vi "StopOnSightProportional.vi"() -> ()   [LabVIEW 2013]
uses:
  <vilib>/Platform/TimedLoop/XDataNode/timing_clust.ctl
  <vilib>/Platform/TimedLoop/XDataNode/nitl_modes.ctl
  <vilib>/Platform/TimedLoop/XDataNode/wakeup.ctl
  <vilib>/Instr/_visa.llb/VISA Configure Serial Port (Instr).vi
  <vilib>/FPGAPlugInAG/sbRIO-9642/niLvFpga_Open_sbRIO-9642.vi
  <vilib>/rvi/interface/common/dynamic/niFpgaDynamicAddResources.vi
  <vilib>/rvi/interface/common/niFpgaWaitOnOcc.vi
  <vilib>/Utility/error.llb/Error Cluster From Error Code.vi
  <vilib>/rvi/errors/niLvFpgaAdjustHostInterfaceError.vi
  <vilib>/Platform/TimedLoop/XDataNode/XDataNode.xnode
  <vilib>/rvi/interface/nirviOpenFPGA/nirviOpenFPGA.xnode
  FPGA Bitfiles/NatesProject1_FPGATarget_FPGAConfig_gDHlPw7zMRU.lvbitx
  FPGA Config.vi
  <vilib>/rvi/interface/nirviReadWriteControl/nirviReadWriteControl.xnode
  <vilib>/Platform/TimedLoop/XDataNode/XDNodeRunTimeDep.lvlib
  NiFpgaLv.dll
  <vilib>/rvi/interface/Simulation/niFpgaSimulationCallBeginRW.vi
panel:
  in  "Stop Distance":dbl(slide) scale=0.1..1.5
  out "error out":errorcluster
  out "Distance\n(cm)":dbl(slide) scale=0.0..1.5
  out "ModA/AI0":fxp<+/-,26,5>
  in  "VISA resource name":refnum<visa-resource-name>
  in  "stop":bool
  out "write buffer":string
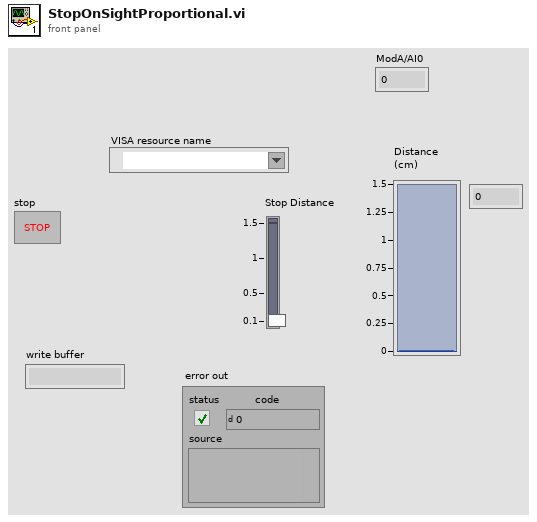
[diagram p1: front panel]
types:
  T1 = typedef "XDNodeRunTimeDep.lvlib/timing_clust.ctl" = cluster{"Expected End [f-1]":u64, "Actual End [f-1]":u64, "Finished Late? [f-1]":bool, "Expected End [i-1]":u64, "Actual End [i-1]":u64, "Finished Late? [i-1]":bool, "Expected Start [i]":u64, "Actual Start [i]":u64, "Expected Start [f]":u64, "Actual Start [f]":u64, "Source Name":string, "Structure Name":string, "Period":i64, "Deadline":i64, "Offset":i64, "Start":i64, "Priority":i32, "Timeout":i32, "Mode":T2, "Wakeup Reason":T3, "Error":errorcluster, "Source Type":string, "Secondary Source Type":string, "Global End Time":u64, "Global Start Time":u64, "Frame Duration":u64, "Iteration Duration":u64, "Assigned CPU":i32, "I/O Scan Engine Mode":u32}
  T2 = typedef "XDNodeRunTimeDep.lvlib/nitl_modes.ctl" = enum32{"No Change", "Process missed periods, maintain original phase", "Discard missed periods, maintain original phase", "Process missed periods, ignore original phase", "Discard missed periods, ignore original phase"}
  T3 = typedef "XDNodeRunTimeDep.lvlib/wakeup.ctl" = enum32{"Normal", "Aborted", "Asynchronous wakeup", "Timing source error", "Timed loop error", "Timeout"}
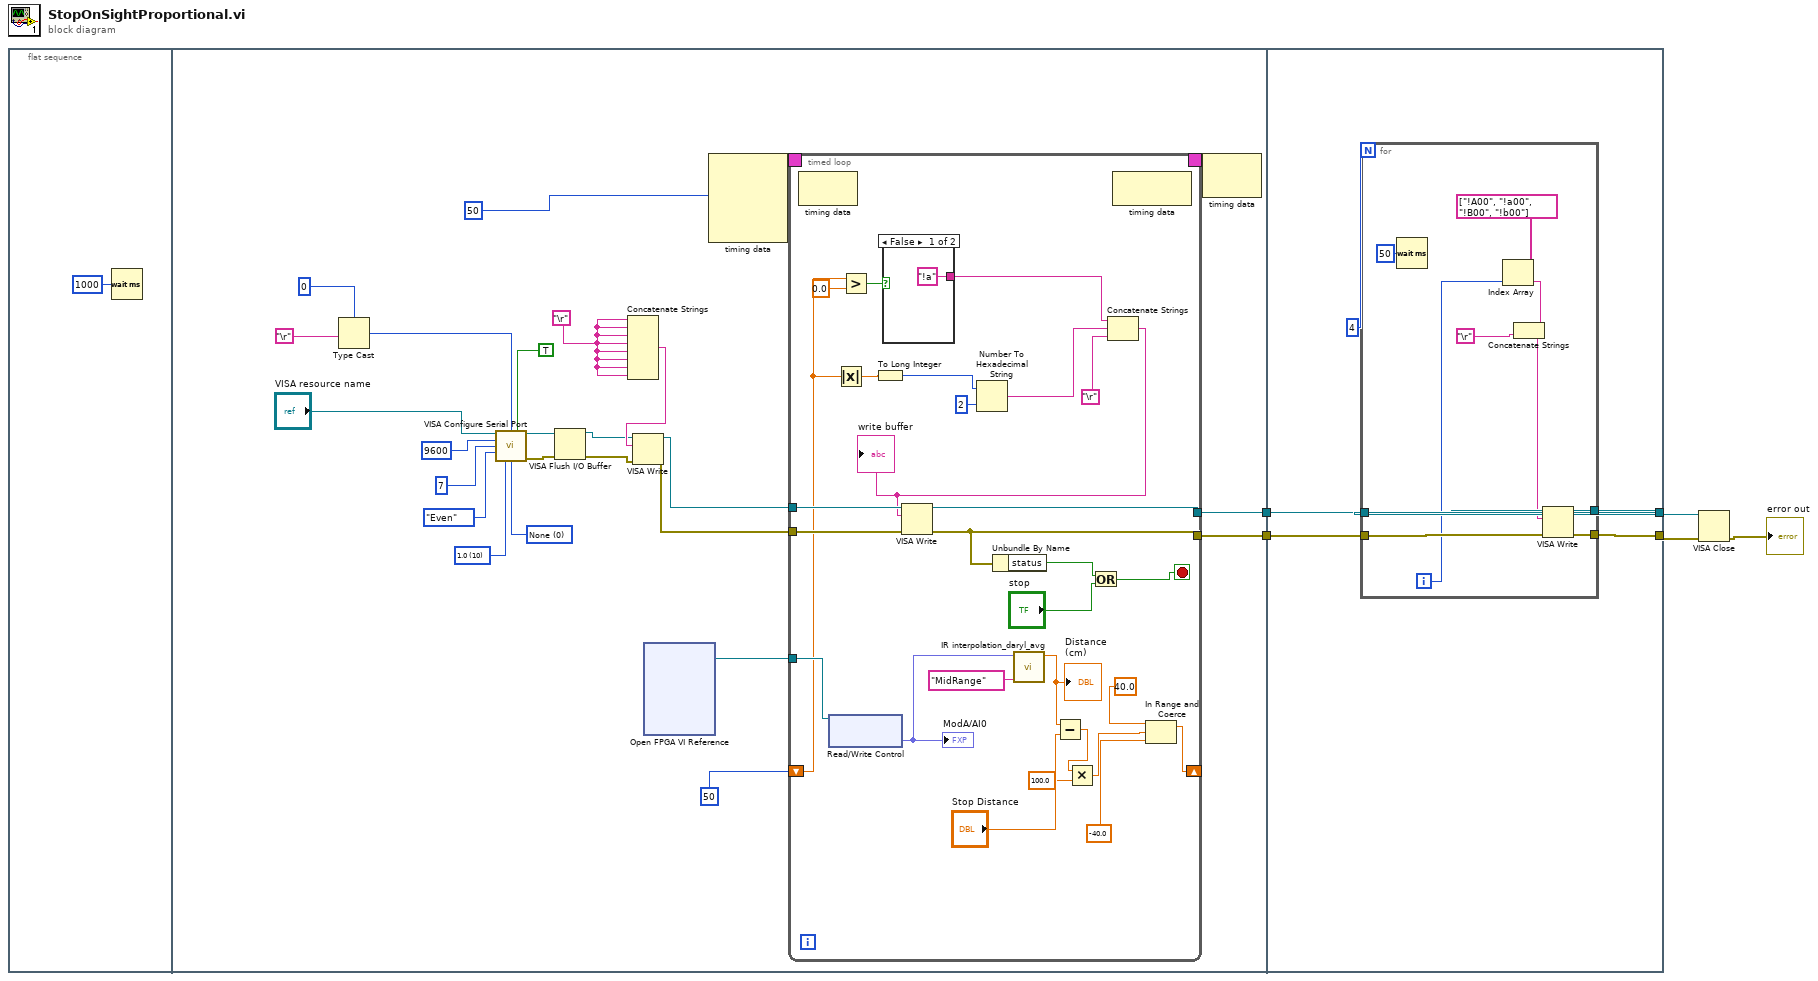
[diagram p0: block diagram]
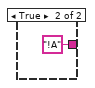
[diagram p2: hidden frame]
diagram:
  n1 = flat-sequence {
    tunnel: [w10] -> w5
    tunnel: [w9] -> w4
    tunnel: [w69] -> w2
    tunnel: [w70] -> w3
    tunnel: w5 -> [w72]
    tunnel: w4 -> [w71]
    frame #0 {
      n2 = Wait (ms)(milliseconds to wait=u32 1000) -> ()  [unwired: 1 out]
    }
    frame #1 {
      w16 = "\r"
      w23 = u16 0 items=["None", "XON/XOFF", "RTS/CTS", "XON/XOFF & RTS/CTS", "DTR/DSR", "XON/XOFF & DTR/DSR"] ("flow control (0:none)")
      w24 = u16 10 items=["1.0"=10, "1.5"=15, "2.0"=20] ("stop bits (10: 1 bit)")
      n3 = Type Cast(type=0, x="\r") -> (*(type *) &x=w19:i32)
      n4 = call-poly "VISA Configure Serial Port"("VISA resource name"="VISA resource name", "termination char\n(0xA = '\\n' = LF)"=w19, "Enable Termination\nChar (T)"=TRUE ("Enable Termination\nChar (T)"), "baud rate (9600)"=u32 9600, "data bits (8)"=u16 7, "parity (0:none)"=enum16{"None", "Odd", "Even", "Mark", "Space"}."Even", "stop bits (10: 1 bit)"=w24, "flow control (0:none)"=w23) -> ("VISA resource name out"=w17:refnum<visa-resource-name>, "error out"=w18:errorcluster)  [unwired: 6 in]
      n5 = VISA Flush I/O Buffer(VISA resource name=w17, error in (no error)=w18) -> (VISA resource name out=w14:refnum<visa-resource-name>, error out=w13:errorcluster)  [unwired: 1 in]
      n6 = Concatenate Strings(w16, w16, w16, w16, w16, w16, w16, w16) -> (w15:string)
      n7 = VISA Write(VISA resource name=w14, write buffer=w15, error in (no error)=w13) -> (VISA resource name out=w12:refnum<visa-resource-name>, error out=w11:errorcluster)  [unwired: 1 out]
      n8 = xnode "Open FPGA VI Reference"() -> ("FPGA VI Reference Out"=w8:refnum<k20>)  [unwired: 2 in, 1 out]
      n9 = node-c288(i64 50 ("Period")) -> (w31:T1)  [unwired: 3 in]
      n10 = timed-loop {
        timing: w31 -> [_]
        timing-out: [_] -> w30
        tunnel: w12 -> [w56]
        tunnel: w11 -> [w55]
        tunnel: [w50] -> w10
        tunnel: [w51] -> w9
        tunnel: w8 -> [w47]
        shift-right: [w42] -> _
        shift-left: 50 -> [w35]
        stop <- w41 stop-if-true
        n11 = node-c288() -> ()  [unwired: 1 in, 1 out]
        n12 = xnode "Read/Write Control"("FPGA VI Reference In"=w47) -> ("ModA/AI0"=w49:fxp<+/-,26,5>)  [unwired: 1 in, 2 out]
        "ModA/AI0" <- w49
        n13 = Absolute Value(x=w35) -> (abs(x)=w36:dbl)
        n14 = Greater?(x=w35, y=0.0) -> (0:w38:bool)
        n15 = To Long Integer(number=w36) -> (32bit integer=w37:i32)
        n16 = case shown="False" w38 {
          tunnel: ["!a" "!A"] -> w40
          frame False {
          }
          frame True {
          }
        }
        n17 = Number To Hexadecimal String(1:i16 2 ("width (-)"), 2:w37) -> (0:w58:string)
        n18 = call "IR interpolation_daryl_avg.vi"("IR Sensor Type"="MidRange", "x value"=w49) -> ("interpolation value"=w45:dbl)  [unwired: 9 in]
        "Distance\n(cm)" <- w45
        n19 = Subtract(x=w45, y="Stop Distance") -> (x-y=w34:dbl)
        n20 = Multiply(x=w34, y=100.0) -> (x*y=w32:dbl)
        n21 = Concatenate Strings(w40, w58, "\r") -> (w54:string)
        "write buffer" <- w54
        n22 = VISA Write(VISA resource name=w56, write buffer=w54, error in (no error)=w55) -> (VISA resource name out=w50:refnum<visa-resource-name>, error out=w51:errorcluster)  [unwired: 1 out]
        n23 = Unbundle By Name(w51) -> ("status"=w53:bool)
        n24 = Or(x=w53, y="stop") -> (x .or. y?=w41:bool)
        n25 = node-c288() -> ()  [unwired: 1 in, 1 out]
        n26 = In Range and Coerce(upper limit=40.0, x=w32, lower limit=-40.0) -> (coerced(x)=w42:dbl)  [unwired: 1 out]
      }
      n27 = node-c288(w30) -> ()  [unwired: 1 out]
    }
    frame #2 {
      n28 = for {
        N: 4 -> [_]
        tunnel: w72 -> [w82]
        tunnel: w71 -> [w81]
        tunnel: [w80] -> w70
        tunnel: [w79] -> w69
        i -> [w77]
        n29 = Wait (ms)(milliseconds to wait=u32 50) -> ()  [unwired: 1 out]
        n30 = Index Array(array=string[] ["!A00", "!a00", "!B00", "!b00"], index=w77) -> (element=w75:string)
        n31 = Concatenate Strings(w75, "\r") -> (w73:string)
        n32 = VISA Write(VISA resource name=w82, write buffer=w73, error in (no error)=w81) -> (VISA resource name out=w80:refnum<visa-resource-name>, error out=w79:errorcluster)  [unwired: 1 out]
      }
    }
  }
  n33 = VISA Close(VISA resource name=w3, error in (no error)=w2) -> (error out=→"error out":errorcluster)
